vi "CCitemTagsList.vi"(8 "error in (no error)":errorcluster) -> (0 "error out":errorcluster, 3 "Array":string[][](array[string]))   [LabVIEW 2013, in "main.lvlib" / "ClearCanvasLibrary.lvlib"]
uses:
  ClearCanvasLibrary.lvlib
  C:/Users/Simon/SkyDrive/LabView/2013/DM2020/DICOM/ClearCanvasNewBuild/ClearCanvas.Dicom.dll
  ClearCanvasNewBuild/ClearCanvas.Dicom.dll
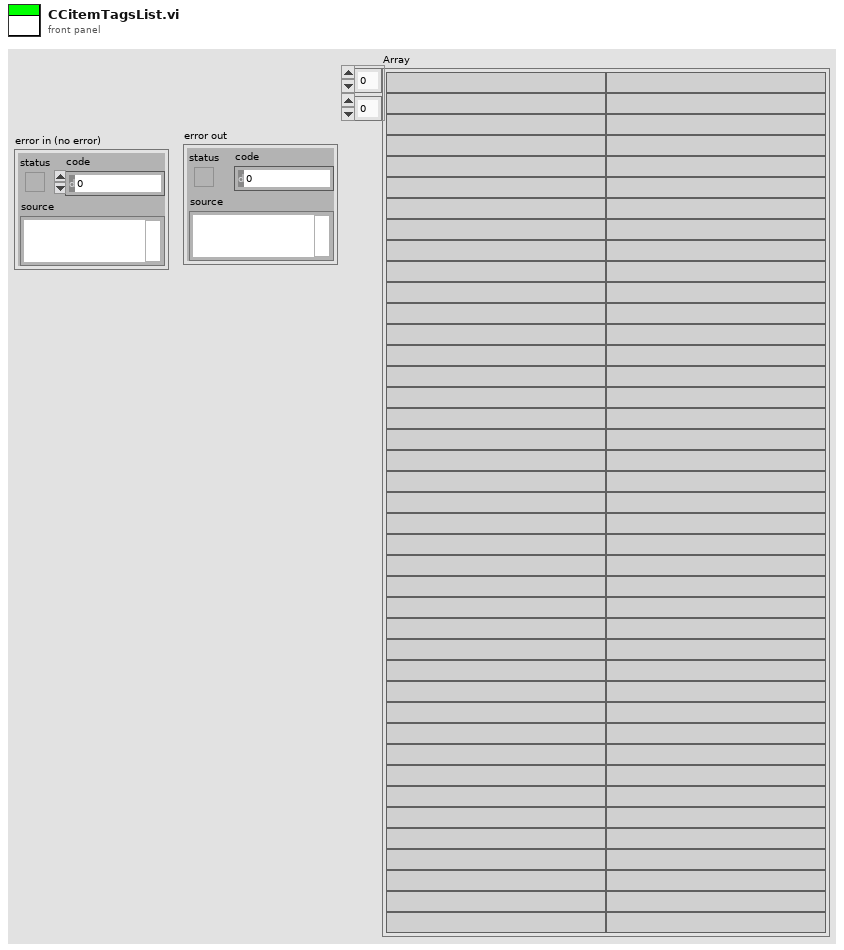
[diagram p1: front panel]
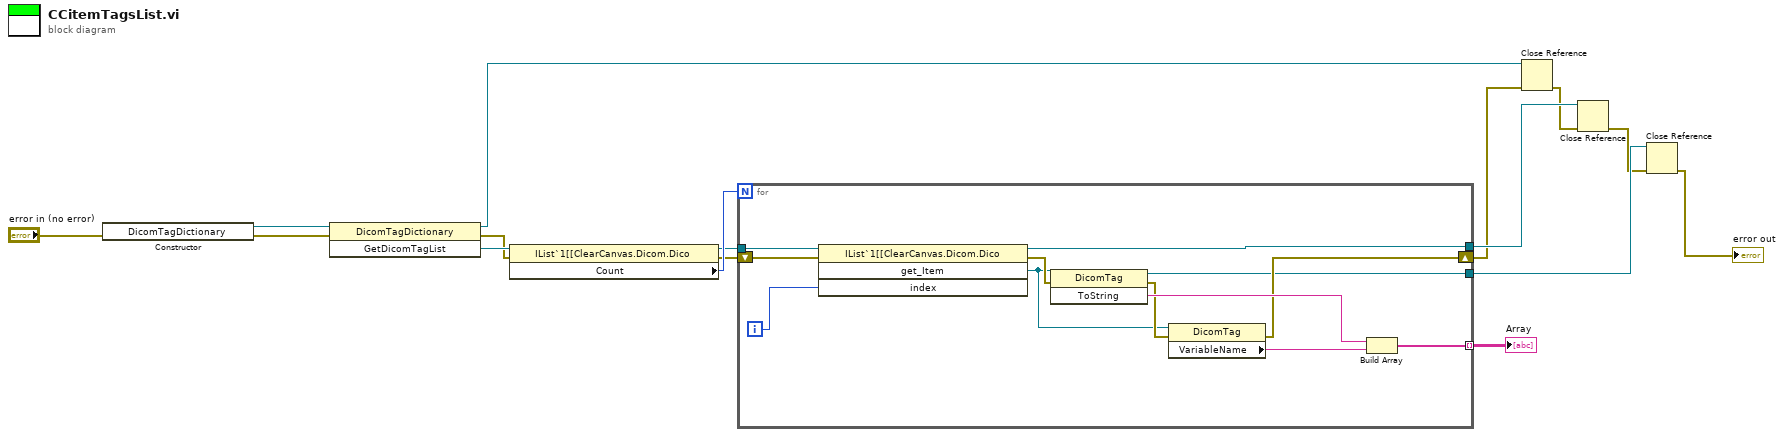
[diagram p0: block diagram]
diagram:
  n1 = constructor class="DicomTagDictionary"(error in="error in (no error)") -> (reference out=w13:refnum<k24>, error out=w16:errorcluster)  [unwired: 2 in, 1 out]
  n2 = invoke class="DicomTagDictionary" method="GetDicomTagList"(reference=w13, error in=w16) -> (reference out=w7:refnum<k24>, error out=w9:errorcluster, "GetDicomTagList"=w15:refnum<k24>)  [unwired: 1 in]
  n3 = property class="IList`1[[ClearCanvas.Dicom.Dico"(reference=w15, error in=w9) -> (reference out=w11:refnum<k24>, error out=w10:errorcluster, "Count"=w14:i32)
  n4 = for {
    N: w14 -> [_]
    tunnel: w11 -> [w28]
    tunnel: [w25] -> w12 mode=indexing
    shift-right: [w20] -> w1
    shift-left: w10 -> [w27]
    tunnel: [w19] -> w6
    tunnel: [w18] -> w5
    i -> [w26]
    n5 = invoke class="IList`1[[ClearCanvas.Dicom.Dico" method="get_Item"(reference=w28, error in=w27, "index"=w26) -> (reference out=w19:refnum<k24>, error out=w22:errorcluster, "get_Item"=w17:refnum<k24>)  [unwired: 1 in, 1 out]
    n6 = invoke class="DicomTag" method="ToString"(reference=w17, error in=w22) -> (reference out=w18:refnum<k24>, error out=w21:errorcluster, "ToString"=w23:string)  [unwired: 1 in]
    n7 = property class="DicomTag"(reference=w17, error in=w21) -> (error out=w20:errorcluster, "VariableName"=w24:string)  [unwired: 1 out]
    n8 = Build Array(w23, w24) -> (w25:string[])
  }
  "Array" <- w12
  n9 = Close Reference(reference=w7, error in (no error)=w1) -> (error out=w4:errorcluster)
  n10 = Close Reference(reference=w6, error in (no error)=w4) -> (error out=w3:errorcluster)
  n11 = Close Reference(reference=w5, error in (no error)=w3) -> (error out=→"error out":errorcluster)
